vi "Combine Result And NAme.vi"(6 "SetParameter":string, 9 "Analysis":T2, 10 "AlgResultName":string[](array[string]), 11 "DataIn":variant) -> (2 "ResultOut":string[][](array[string]))   [LabVIEW 2019]
uses:
  Analysis/Controls/V_Analysis_Type.ctl
  Analysis/Controls/ShapeDectect/V_ShapeDectectFinalResult.ctl
  Analysis/Controls/Color Pattern Match/Analysis Color Pattern Match Result.ctl
  Analysis/Controls/Geometric Match/Analysis_GeomatricPatternMatch_Result.ctl
  <vilib>/vision/Pattern Matching.llb/IMAQ GM Match Report.ctl
  Ctrl/ROIDataType.ctl
  Analysis/Controls/ShapeDectect/V_ShapeDectectResult.ctl
  Analysis/Controls/ShapeDectect/Analysis_ShapeDectect_Parameter.ctl
  Analysis/Controls/Area Check/Area Check_Result.ctl
  2f9eb778-ec5f-4e43-985a-d17594ea7075.vi
  <vilib>/JDP Science/JSONtext/JSON text to Variant.vi
panel:
  in  "Shapedectect Result Out":T1
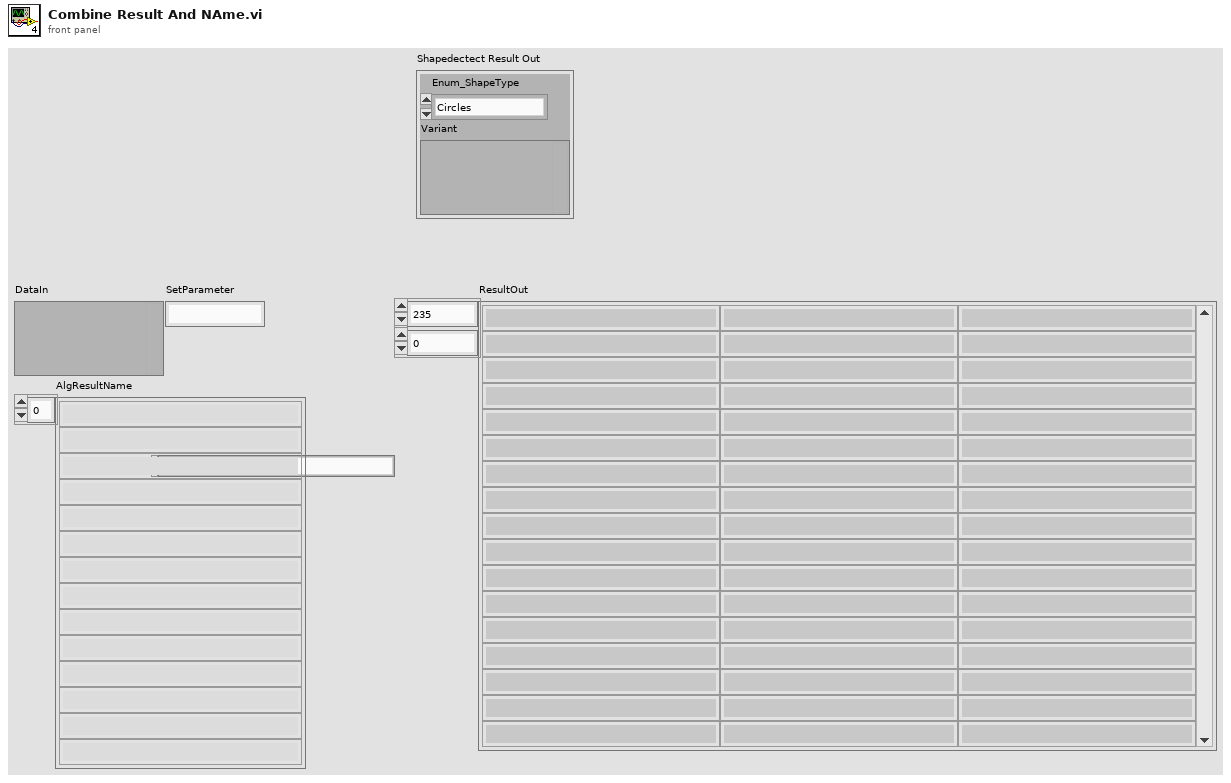
[diagram p1: front panel]
types:
  T1 = typedef "V_ShapeDectectFinalResult.ctl" = cluster{"Enum_ShapeType":enum16{"Circles", "Ellipses", "Lines", "Rectangles"}, "Variant":variant}
  T2 = typedef "V_Analysis_Type.ctl" = enum16{"None", "C_Color Pattern Matching", "G_PatternMatching", "G_ShapeDectect", "G_GeometricMatch", "B_Area Check"}
  T3 = typedef "Analysis Color Pattern Match Result.ctl" = cluster{"Number of Matches":i32, "Matches out":cluster{"Position":cluster{"x":sgl, "y":sgl}, "Angle":sgl, "Scale":sgl, "Score":sgl, "Bounding Box":cluster{"x":sgl, "y":sgl}[]}[], "Calibrated Matches":cluster{"Position":cluster{"x":sgl, "y":sgl}, "Angle":sgl, "Scale":sgl, "Score":sgl, "Bounding Box":cluster{"x":sgl, "y":sgl}[]}[], "ROI Descriptor":T4, "ROIName":string}
  T4 = typedef "ROI Descriptor" = cluster{"Global Rectangle":i32[], "Contours":cluster{"ID":enum32{"External", "Internal"}, "Type":u32, "Coordinates":i32[]}[]}
  T5 = typedef "Analysis_ShapeDectect_Parameter.ctl" = cluster{"Enum_ShapeType":enum16{"Circles", "Ellipses", "Lines", "Rectangles"}, "MaxParticle":i32, "Descriptor":cluster{"Set 1":dbl, "Set 2":dbl, "Set 3":dbl, "Set 4":dbl}, "Match Options":cluster{"Rotation":bool, "Scale":bool, "Occlusion":bool, "Range Settings":cluster{"Match Constraints":u32, "Min":dbl, "Max":dbl}[]}, "Curve Parameters":cluster{"Extraction Mode":u32, "Edge Threshold":i32, "Edge Filter Size":u32, "Min Length":i32, "Row Search Step Size":i32, "Col Search Step Size":i32, "Max Endpoint Gap":i32, "Closed":bool, "Subpixel":bool}, " score":dbl}
  T6 = typedef "Area Check_Result.ctl" = cluster{"AreaDataOut":cluster{"AreaDataOut":cluster{"Rectangle":T7, "Particle Measurements (Pixels)":dbl[][]}}[], "Percent":dbl[], "Item?":bool, "ROI":i32[]}
  T7 = typedef "IMAQ Rectangle" = cluster{"Left":i32, "Top":i32, "Right":i32, "Bottom":i32, "Rotation":dbl}
  T8 = cluster{"Position":cluster{"x":sgl, "y":sgl}, "Angle":sgl, "Scale":sgl, "Score":sgl, "Bounding Box":cluster{"x":sgl, "y":sgl}[]}[]
  T9 = typedef "Analysis_GeomatricPatternMatch_Result.ctl" = cluster{"Number of Matches":i32, "Matches (pixel)":T10[], "Matches (real-world)":T10[], "Data out":T11, "ROIName":string}
  T10 = typedef "IMAQ GM Match Report.ctl" = cluster{"Position":cluster{"x":sgl, "y":sgl}, "Angle":sgl, "Scale":sgl, "Score":sgl, "Bounding Box":cluster{"x":sgl, "y":sgl}[], "Contrast Reversed":bool, "Occlusion %":sgl, "Template Target Curve Score":sgl, "Target Template Curve Score":sgl, "Correlation Score":sgl}
  T11 = typedef "ROIDataType.ctl" = cluster{"Global Rectangle":i32[], "Contours":cluster{"Contour Type":u32, "ROI Type":u32, "Points":i32[]}[]}
  T12 = typedef "V_ShapeDectectResult.ctl" = cluster{"ResultOut":variant, "DectectItem":i32, "Data out":T11, "ROIName":string}
  T13 = enum16{"Circles", "Ellipses", "Lines", "Rectangles"}
  T14 = cluster{"Index":string[], "DectectData":string[]}
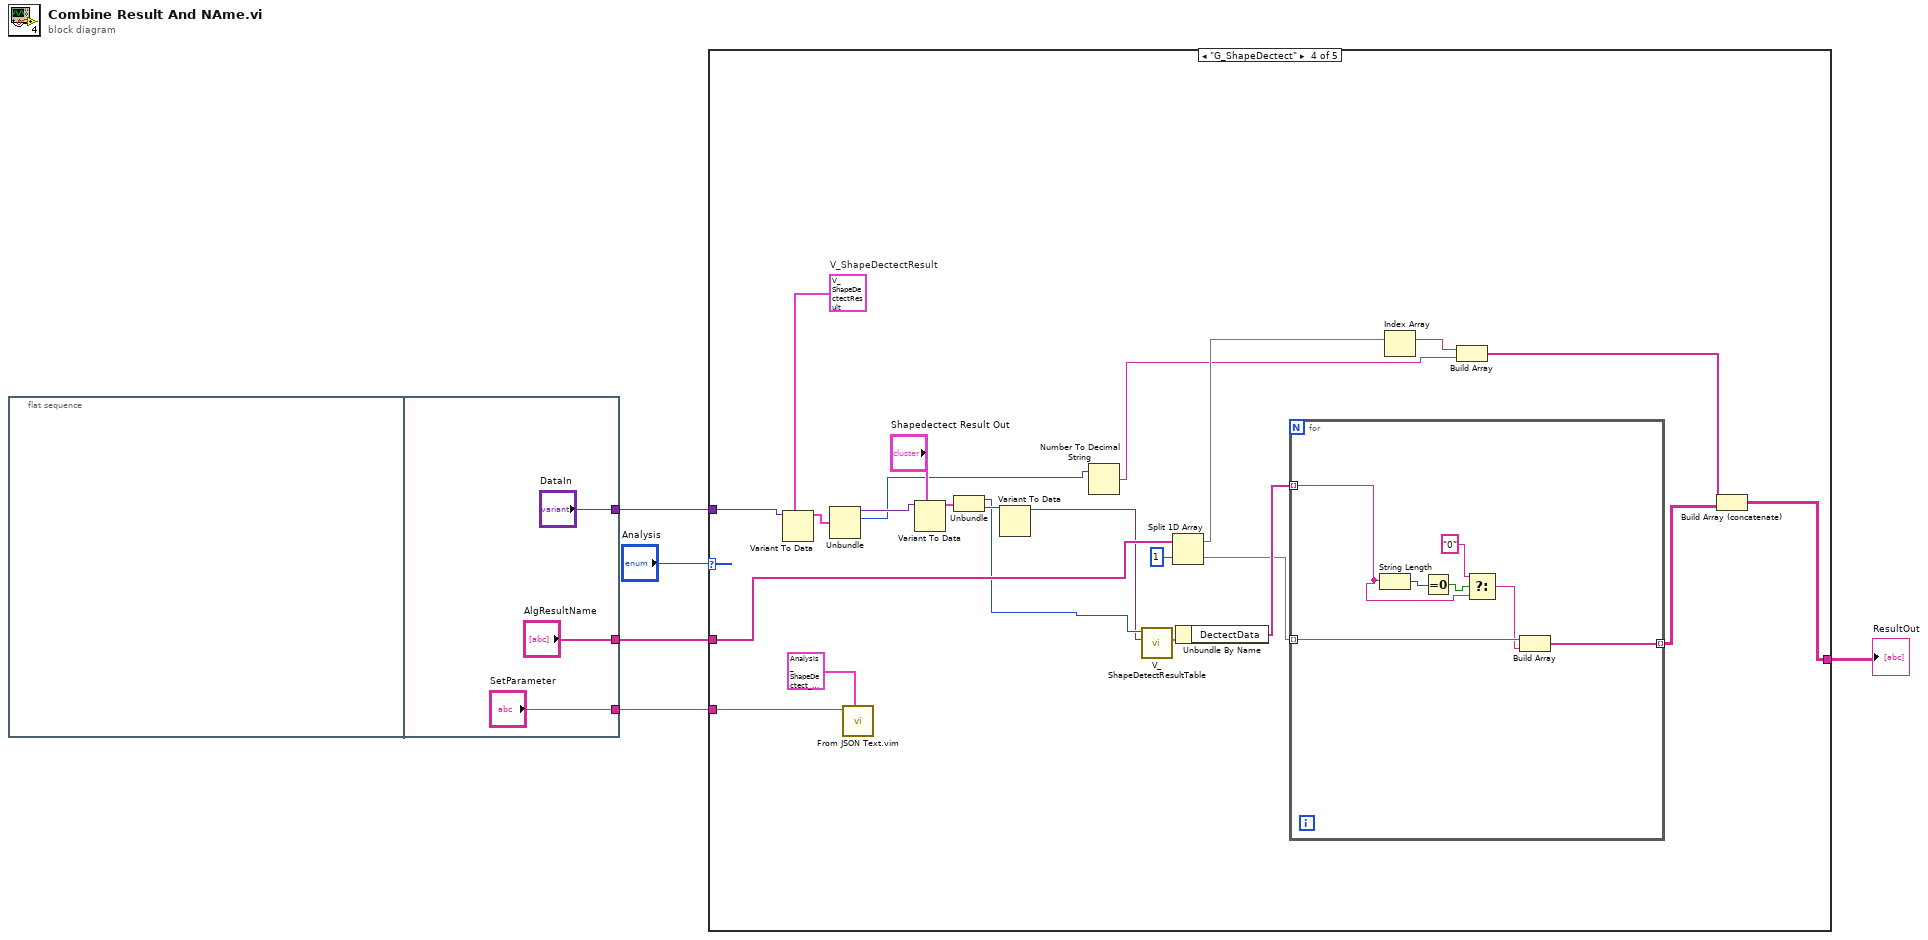
[diagram p0: block diagram]
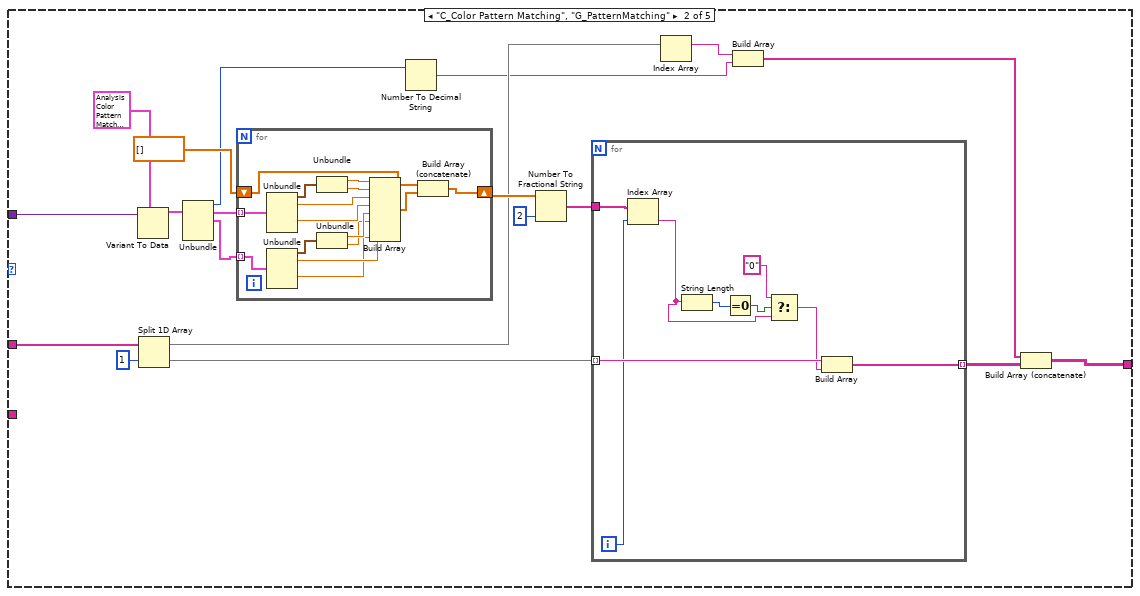
[diagram p3: hidden frame]
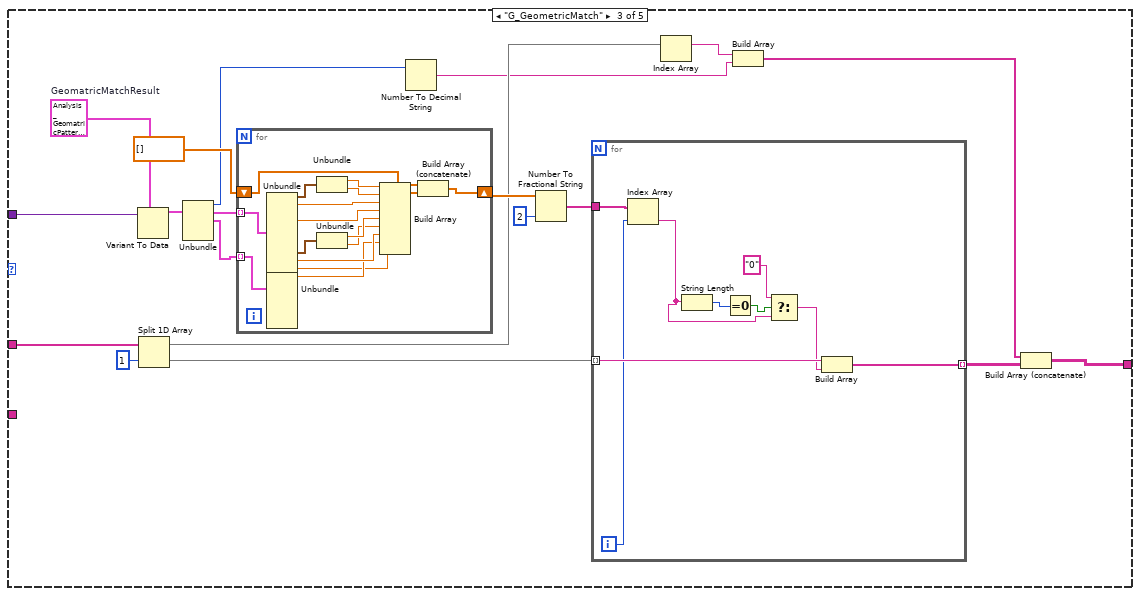
[diagram p4: hidden frame]
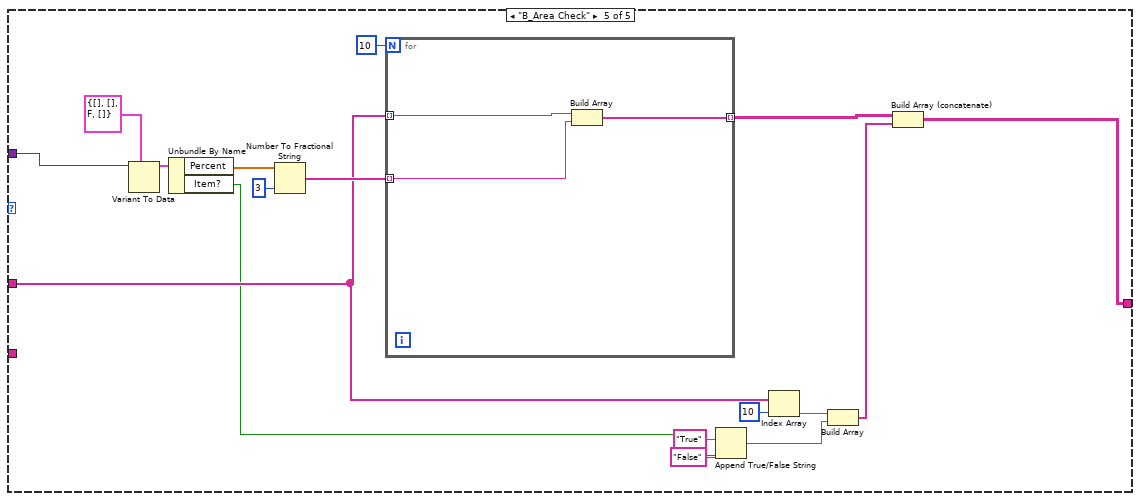
[diagram p5: hidden frame]
diagram:
  n1 = flat-sequence {
    tunnel: ["DataIn"] -> w5
    tunnel: ["AlgResultName"] -> w4
    tunnel: ["SetParameter"] -> w1
    frame #0 {
    }
    frame #1 {
    }
  }
  n2 = case shown="\"G_ShapeDectect\"" "Analysis" {
    tunnel: w5 -> [_ w27 w70 w101 w142]
    tunnel: w4 -> [_ w24 w67 w115 w135]
    tunnel: [_ w15 w58 w106 w126] -> w3
    tunnel: w1 -> [_ _ _ w117 _]
    frame "None", Default {
    }
    frame "C_Color Pattern Matching", "G_PatternMatching" {
      n3 = Variant To Data(type=T3 {"Number of Matches"=0, "Matches out"=[{"Position"={"x"=123.0, "y"=0.0}, "Angle"=0.0, "Scale"=0.0, "Score"=0.0, "Bounding Box"=[]}, {"Position"={"x"=0.0, "y"=0.0}, "Angle"=0.0, "Scale"=0.0, "Score"=0.0, "Bounding Box"=[]}, {"Position"={"x"=0.0, "y"=0.0}, "Angle"=0.0, "Scale"=0.0, "Score"=0.0, "Bounding Box"=[]}, {"Position"={"x"=444.0, "y"=0.0}, "Angle"=0.0, "Scale"=0.0, "Score"=0.0, "Bounding Box"=[]}], "Calibrated Matches"=[], "ROI Descriptor"={"Global Rectangle"=[], "Contours"=[]}, "ROIName"=""} ("Color Pattern Matching"), Variant=w27) -> (data=w25:T3)  [unwired: 1 in, 1 out]
      n4 = Split 1D Array(array=w24, index=1) -> (first subarray=w14:string[], second subarray=w22:string[])
      n5 = Unbundle(w25) -> ("Number of Matches"=w12:i32, "Matches out"=w21:T8, "Calibrated Matches"=w9:T8)  [unwired: 2 out]
      n6 = for {
        tunnel: w21 -> [w41] mode=indexing
        shift-right: [w34] -> w20
        shift-left: sgl[] [] -> [w35]
        tunnel: w9 -> [w32] mode=indexing
        n7 = Unbundle(w41) -> ("Position"=w42:cluster{"x":sgl, "y":sgl}, "Angle"=w38:sgl, "Score"=w37:sgl)  [unwired: 2 out]
        n8 = Unbundle(w32) -> ("Position"=w33:cluster{"x":sgl, "y":sgl}, "Angle"=w29:sgl, "Score"=w28:sgl)  [unwired: 2 out]
        n9 = Unbundle(w42) -> ("x"=w40:sgl, "y"=w39:sgl)
        n10 = Unbundle(w33) -> ("x"=w31:sgl, "y"=w30:sgl)
        n11 = Build Array(w40, w39, w38, w37, w31, w30, w29, w28) -> (w36:sgl[])
        n12 = Build Array (concatenate)(w35, w36) -> (w34:sgl[])
      }
      n13 = Number To Decimal String(number=w12) -> (decimal integer string=w11:string)  [unwired: 1 in]
      n14 = Number To Fractional String(number=w20, precision (6)=i16 2) -> (F-format string=w18:string[])  [unwired: 2 in]
      n15 = for {
        tunnel: w22 -> [w51] mode=indexing
        tunnel: w18 -> [w50]
        tunnel: [w48] -> w16 mode=indexing
        i -> [w49]
        n16 = Index Array(array=w50, index=w49) -> (element=w45:string)
        n17 = String Length(string=w45) -> (length=w47:i32)
        n18 = Equal To 0?(x=w47) -> (x = 0?=w46:bool)
        n19 = Select(t="0", s=w46, f=w45) -> (s? t:f=w44:string)
        n20 = Build Array(w51, w44) -> (w48:string[])
      }
      n21 = Index Array(array=w14) -> (element=w13:string)  [unwired: 1 in]
      n22 = Build Array(w13, w11) -> (w10:string[])
      n23 = Build Array (concatenate)(w10, w16) -> (w15:string[][])
    }
    frame "G_GeometricMatch" {
      w69 = T9 {"Number of Matches"=0, "Matches (pixel)"=[{"Position"={"x"=123.0, "y"=0.0}, "Angle"=0.0, "Scale"=0.0, "Score"=0.0, "Bounding Box"=[], "Contrast Reversed"=FALSE, "Occlusion %"=0.0, "Template Target Curve Score"=0.0, "Target Template Curve Score"=0.0, "Correlation Score"=0.0}, {"Position"={"x"=0.0, "y"=0.0}, "Angle"=0.0, "Scale"=0.0, "Score"=0.0, "Bounding Box"=[], "Contrast Reversed"=FALSE, "Occlusion %"=0.0, "Template Target Curve Score"=0.0, "Target Template Curve Score"=0.0, "Correlation Score"=0.0}, {"Position"={"x"=0.0, "y"=0.0}, "Angle"=0.0, "Scale"=0.0, "Score"=0.0, "Bounding Box"=[], "Contrast Reversed"=FALSE, "Occlusion %"=0.0, "Template Target Curve Score"=0.0, "Target Template Curve Score"=0.0, "Correlation Score"=0.0}, {"Position"={"x"=444.0, "y"=0.0}, "Angle"=0.0, "Scale"=0.0, "Score"=0.0, "Bounding Box"=[], "Contrast Reversed"=FALSE, "Occlusion %"=0.0, "Template Target Curve Score"=0.0, "Target Template Curve Score"=0.0, "Correlation Score"=0.0}], "Matches (real-world)"=[], "Data out"={"Global Rectangle"=[], "Contours"=[]}, "ROIName"=""}  # GeomatricMatchResult
      n24 = Variant To Data(type=w69, Variant=w70) -> (data=w68:T9)  [unwired: 1 in, 1 out]
      n25 = Split 1D Array(array=w67, index=1) -> (first subarray=w57:string[], second subarray=w65:string[])
      n26 = Unbundle(w68) -> ("Number of Matches"=w55:i32, "Matches (pixel)"=w64:T10[], "Matches (real-world)"=w52:T10[])  [unwired: 2 out]
      n27 = for {
        tunnel: w64 -> [w85] mode=indexing
        shift-right: [w78] -> w63
        shift-left: sgl[] [] -> [w79]
        tunnel: w52 -> [w76] mode=indexing
        n28 = Unbundle(w85) -> ("Position"=w86:cluster{"x":sgl, "y":sgl}, "Angle"=w82:sgl, "Score"=w81:sgl)  [unwired: 7 out]
        n29 = Unbundle(w76) -> ("Position"=w77:cluster{"x":sgl, "y":sgl}, "Angle"=w73:sgl, "Scale"=w71:sgl, "Score"=w72:sgl)  [unwired: 6 out]
        n30 = Unbundle(w86) -> ("x"=w84:sgl, "y"=w83:sgl)
        n31 = Unbundle(w77) -> ("x"=w75:sgl, "y"=w74:sgl)
        n32 = Build Array(w84, w83, w82, w81, w75, w74, w73, w72, w71) -> (w80:sgl[])
        n33 = Build Array (concatenate)(w79, w80) -> (w78:sgl[])
      }
      n34 = Number To Decimal String(number=w55) -> (decimal integer string=w54:string)  [unwired: 1 in]
      n35 = Number To Fractional String(number=w63, precision (6)=i16 2) -> (F-format string=w61:string[])  [unwired: 2 in]
      n36 = for {
        tunnel: w65 -> [w95] mode=indexing
        tunnel: w61 -> [w94]
        tunnel: [w92] -> w59 mode=indexing
        i -> [w93]
        n37 = Index Array(array=w94, index=w93) -> (element=w89:string)
        n38 = String Length(string=w89) -> (length=w91:i32)
        n39 = Equal To 0?(x=w91) -> (x = 0?=w90:bool)
        n40 = Select(t="0", s=w90, f=w89) -> (s? t:f=w88:string)
        n41 = Build Array(w95, w88) -> (w92:string[])
      }
      n42 = Index Array(array=w57) -> (element=w56:string)  [unwired: 1 in]
      n43 = Build Array(w56, w54) -> (w53:string[])
      n44 = Build Array (concatenate)(w53, w59) -> (w58:string[][])
    }
    frame "G_ShapeDectect" {
      w100 = T12 {"ResultOut"=variant, "DectectItem"=0, "Data out"={"Global Rectangle"=[], "Contours"=[]}, "ROIName"=""}  # V_ShapeDectectResult
      n45 = Variant To Data(type=w100, Variant=w101) -> (data=w99:T12)  [unwired: 1 in, 1 out]
      n46 = Unbundle(w99) -> ("ResultOut"=w98:variant, "DectectItem"=w96:i32)  [unwired: 2 out]
      n47 = call "From JSON Text.vim"("Data Type and Default Value"=T5 {"Enum_ShapeType"=enum."Circles", "MaxParticle"=1, "Descriptor"={"Set 1"=100.0, "Set 2"=10.0, "Set 3"=200.0, "Set 4"=10.0}, "Match Options"={"Rotation"=TRUE, "Scale"=FALSE, "Occlusion"=FALSE, "Range Settings"=[{"Match Constraints"=0, "Min"=0.0, "Max"=360.0}]}, "Curve Parameters"={"Extraction Mode"=0, "Edge Threshold"=75, "Edge Filter Size"=1, "Min Length"=25, "Row Search Step Size"=15, "Col Search Step Size"=15, "Max Endpoint Gap"=10, "Closed"=FALSE, "Subpixel"=FALSE}, " score"=500.0} ("SetParameter"), "JSON"=w117) -> ()  [unwired: 8 in, 2 out]
      n48 = Variant To Data(type="Shapedectect Result Out", Variant=w98) -> (data=w104:T1)  [unwired: 1 in, 1 out]
      n49 = Unbundle(w104) -> ("Enum_ShapeType"=w102:T13, "Variant"=w103:variant)
      n50 = Variant To Data(Variant=w103) -> (data=w97:variant)  [unwired: 2 in, 1 out]
      n51 = Number To Decimal String(number=w96) -> (decimal integer string=w112:string)  [unwired: 1 in]
      n52 = call "V_ShapeDetectResultTable.vi"("Result"=w97, "Shape Type"=w102) -> ("Result"=w110:T14)  [unwired: 8 in, 1 out]
      n53 = Split 1D Array(array=w115, index=1) -> (first subarray=w113:string[], second subarray=w108:string[])
      n54 = Unbundle By Name(w110) -> ("DectectData"=w109:string[])
      n55 = for {
        tunnel: w108 -> [w125] mode=indexing
        tunnel: w109 -> [w119] mode=indexing
        tunnel: [w124] -> w107 mode=indexing
        n56 = String Length(string=w119) -> (length=w123:i32)
        n57 = Equal To 0?(x=w123) -> (x = 0?=w122:bool)
        n58 = Select(t="0", s=w122, f=w119) -> (s? t:f=w121:string)
        n59 = Build Array(w125, w121) -> (w124:string[])
      }
      n60 = Index Array(array=w113) -> (element=w114:string)  [unwired: 1 in]
      n61 = Build Array(w114, w112) -> (w111:string[])
      n62 = Build Array (concatenate)(w111, w107) -> (w106:string[][])
    }
    frame "B_Area Check" {
      n63 = Variant To Data(type=T6 {"AreaDataOut"=[], "Percent"=[], "Item?"=FALSE, "ROI"=[]} ("cluster"), Variant=w142) -> (data=w140:T6)  [unwired: 1 in, 1 out]
      n64 = Unbundle By Name(w140) -> ("Percent"=w139:dbl[], "Item?"=w131:bool)
      n65 = Number To Fractional String(number=w139, precision (6)=i16 3) -> (F-format string=w137:string[])  [unwired: 2 in]
      n66 = for {
        N: 10 -> [_]
        tunnel: w135 -> [w145] mode=indexing
        tunnel: w137 -> [w144] mode=indexing
        tunnel: [w143] -> w133 mode=indexing
        n67 = Build Array(w145, w144) -> (w143:string[])
      }
      n68 = Append True/False String(1:w131, 2:"False" ("false string"), 3:"True" ("true string")) -> (0:w130:string)  [unwired: 1 in]
      n69 = Index Array(array=w135, index=10) -> (element=w132:string)
      n70 = Build Array(w132, w130) -> (w127:string[])
      n71 = Build Array (concatenate)(w133, w127) -> (w126:string[][])
    }
  }
  "ResultOut" <- w3
